vi "ExecuteMenuCommand.vi"(0 "reference":refnum<class "PackageNode.lvclass">, 1 "Command":string, 5 "error in (no error)":errorcluster) -> (14 "reference out":refnum<class "PackageNode.lvclass">, 15 "EditorAction":T3, 16 "FlattenCommandSettings":T1, 19 "error out":errorcluster)   [LabVIEW 2020, in "PackageNode.lvclass"]
uses:
  <resource>/Framework/Providers/Open_GDS/UML/PackageNode_class/PackageNode.lvclass
  C:/Program Files (x86)/National Instruments/LabVIEW 2020/resource/Framework/Providers/Open_GDS/UML/RectangularNode_class/RectangularNode.lvclass
  C:/Program Files (x86)/National Instruments/LabVIEW 2020/resource/Framework/Providers/Open_GDS/UML/AbstractNode_class/AbstractNode.lvclass
  <resource>/Framework/Providers/Open_GDS/UML/UMLEditor/UMLEditor EditorActionType.ctl
  <resource>/Framework/Providers/Open_GDS/UML/UMLEditor/UMLEditor FlattenCommandType.ctl
  <resource>/Framework/Providers/Open_GDS/UML/UMLEditor/UMLEditor ExecuteCommandType.ctl
  <resource>/Framework/Providers/Open_GDS/UML/General/Rectangle/Rectangle Rectangle2D.ctl
  <resource>/Framework/Providers/Open_GDS/UML/AbstractNode_class/AbstractNode.lvclass
  <resource>/Framework/Providers/Open_GDS/UML/RectangularNode_class/RectangularNode.lvclass
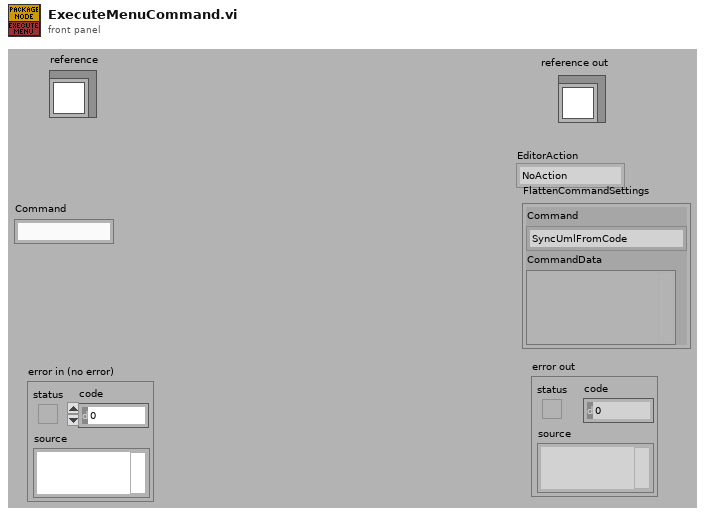
[diagram p1: front panel]
types:
  T1 = typedef "UMLEditor FlattenCommandType.ctl" = cluster{"Command":T2, "CommandData":variant}
  T2 = typedef "UMLEditor ExecuteCommandType.ctl" = enum16{"SyncUmlFromCode", "SyncCodeFromUML", "OpenClass", "OpenFile", "CreateClass", "CreateVI", "OpenClassAttribute", "LocateInProject", "GraphExecute"}
  T3 = typedef "UMLEditor EditorActionType.ctl" = enum16{"NoAction", "Repaint", "ExecuteCommand"}
  T4 = typedef "Rectangle Rectangle2D.ctl" = cluster{"x":dbl, "y":dbl, "width":dbl, "height":dbl}
  T5 = typedef "PackageNode.lvclass/ObjectAttributes.ctl" = cluster{"name":string, "contents":refnum<class "MultiLineString.lvclass">, "DEFAULT_TOP_WIDTH":i32, "DEFAULT_TOP_HEIGHT":i32, "DEFAULT_WIDTH":i32, "DEFAULT_HEIGHT":i32, "NAME_GAP":i32, "XGAP":i32, "YGAP":i32, "Collapsed":bool, "Note color":u32, "Justification":u16}
  T6 = typedef "AbstractNode.lvclass/ObjectAttributes.ctl" = cluster{"parent":refnum<class "AbstractNode.lvclass">, "children":refnum<class "AbstractNode.lvclass">[], "Hidden":bool}
  T7 = typedef "RectangularNode.lvclass/ObjectAttributes.ctl" = cluster{"bounds":T4}
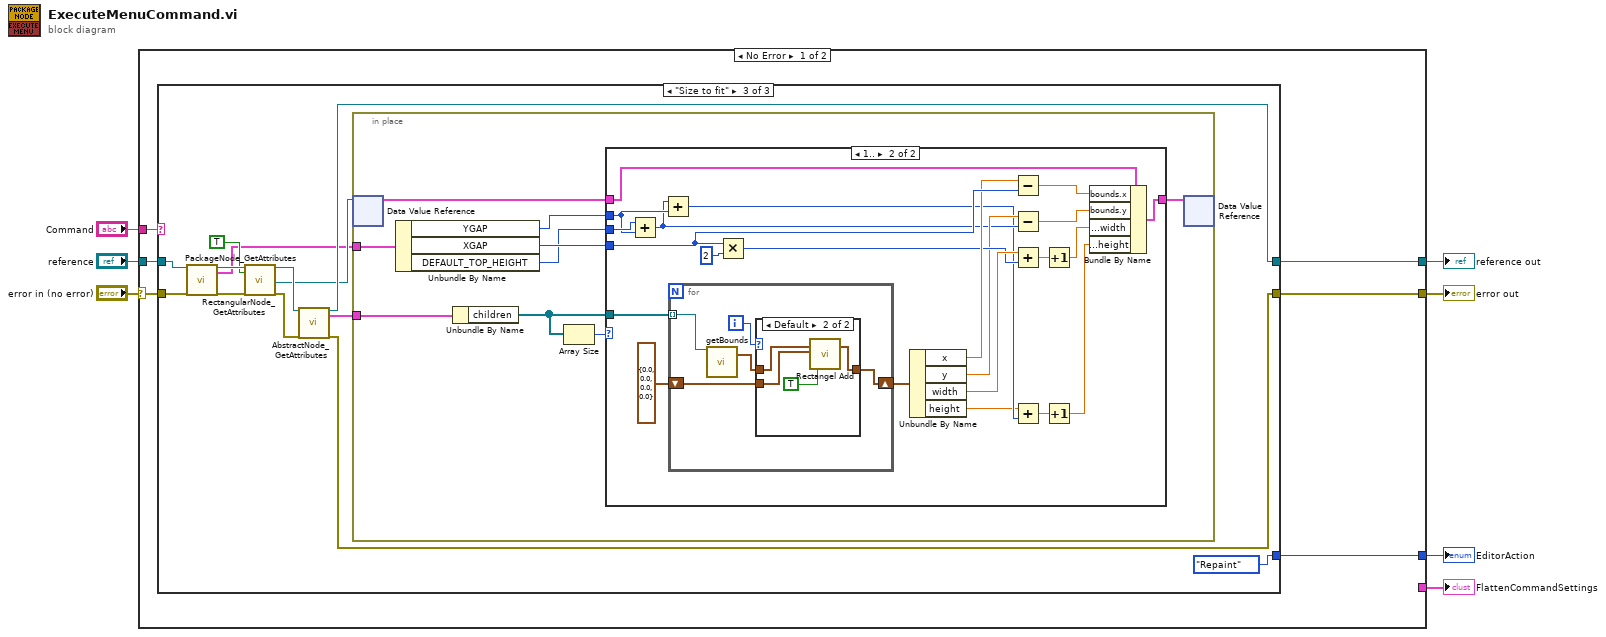
[diagram p0: block diagram]
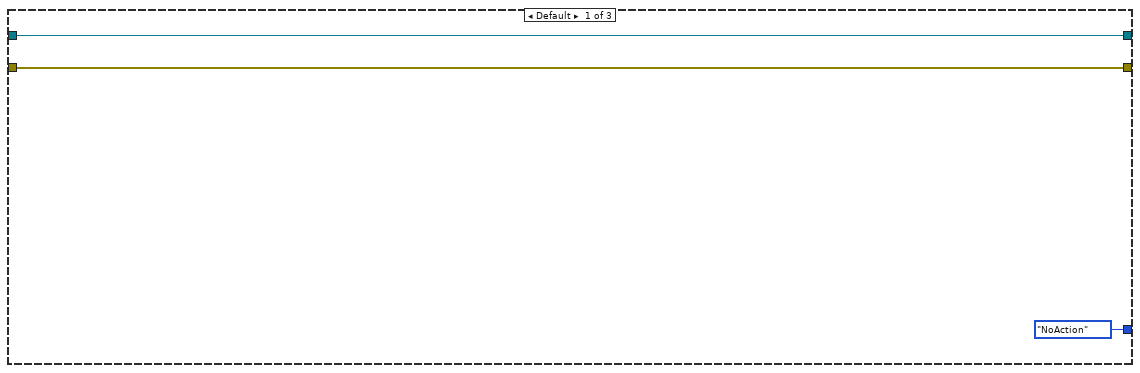
[diagram p2: hidden frame]
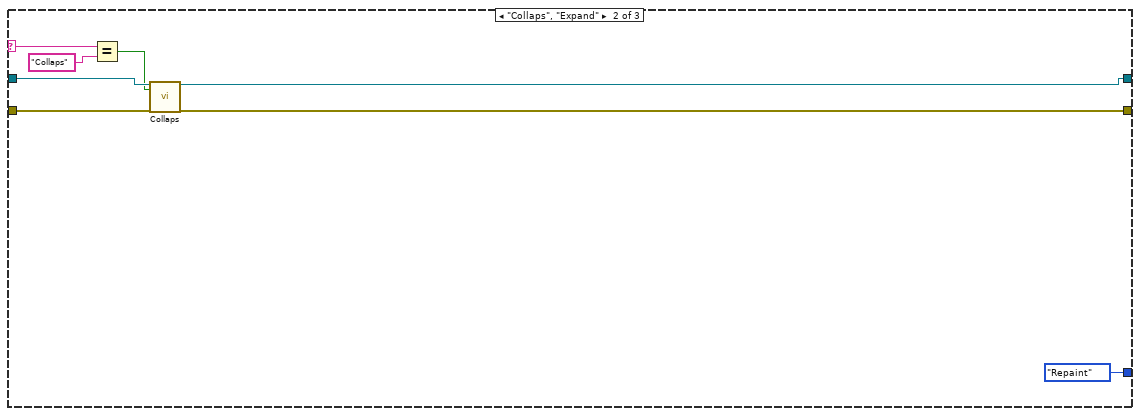
[diagram p3: hidden frame]
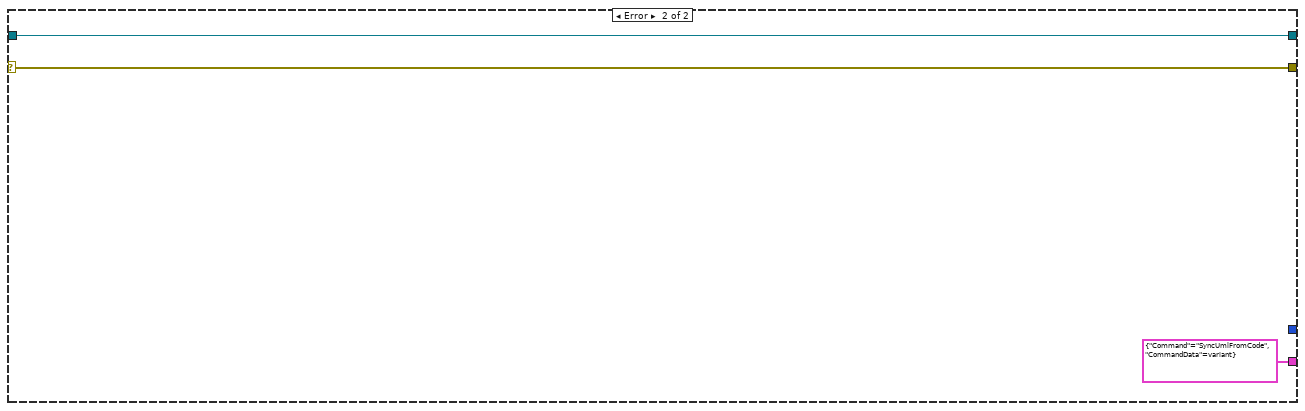
[diagram p6: hidden frame]
diagram:
  n1 = case shown="No Error" "error in (no error)" {
    selector: "error in (no error)" -> [w8 w81]
    tunnel: "reference" -> [w9 w82]
    tunnel: [w11 w81] -> w5
    tunnel: [w12 w82] -> w4
    tunnel: "Command" -> [w13 _]
    tunnel: [w10 _] -> w2
    tunnel: [_ T1 {"Command"=enum."SyncUmlFromCode", "CommandData"=variant} ("FlattenCommandSettings")] -> w1
    frame No Error {
      n2 = case shown="\"Size to fit\"" w13 {
        selector: w13 -> [_ w23 _]
        tunnel: w8 -> [w15 w19 w35]
        tunnel: w9 -> [w16 w21 w37]
        tunnel: [w16 w17 w36] -> w12
        tunnel: [w15 w18 w34] -> w11
        tunnel: [UMLEditor_EditorActionType."NoAction" ("EditorAction") UMLEditor_EditorActionType."Repaint" ("EditorAction") UMLEditor_EditorActionType."Repaint" ("EditorAction")] -> w10
        frame Default {
        }
        frame "Collaps", "Expand" {
          n3 = Equal?(x=w23, y="Collaps") -> (x = y?=w20:bool)
          n4 = call-dynamic "Collaps.vi"("reference in"=w21, "Collaps"=w20, "error in (no error)"=w19) -> ("reference out"=w17:refnum<class "PackageNode.lvclass">, "error out"=w18:errorcluster)  [unwired: 15 in]
        }
        frame "Size to fit" {
          n5 = call <resource>:"PackageNode_GetAttributes.vi"("reference in"=w37, "error in (no error)"=w35) -> ("reference out"=w32:refnum<class "PackageNode.lvclass">, "Data"=w25:T5, "error out"=w31:errorcluster)  [unwired: 14 in, 1 out]
          n6 = call <resource>:"RectangularNode_GetAttributes.vi"("reference in"=w32, "OnlyGetDvrReference(False)"=TRUE, "error in (no error)"=w31) -> ("reference out"=w30:refnum<class "PackageNode.lvclass">, "DataRef"=w28:refnum<data-value>, "error out"=w29:errorcluster)  [unwired: 13 in, 1 out]
          n7 = call <resource>:"AbstractNode_GetAttributes.vi"("reference in"=w30, "error in (no error)"=w29) -> ("reference out"=w36:refnum<class "PackageNode.lvclass">, "Data"=w26:T6, "error out"=w34:errorcluster)  [unwired: 14 in, 1 out]
          n8 = in-place {
            in-place-border: w26 -> [w41]
            in-place-border: w25 -> [w40]
            n9 = in-place-dvr #1(w28) -> (w43:T7)  [unwired: 1 out]
            n10 = Unbundle By Name(w40) -> ("YGAP"=w46:i32, "XGAP"=w45:i32, "DEFAULT_TOP_HEIGHT"=w44:i32)
            n11 = Unbundle By Name(w41) -> ("children"=w39:refnum<class "AbstractNode.lvclass">[])
            n12 = Array Size(array=w39) -> (size(s)=w38:i32)
            n13 = case shown="1.." w38 {
              tunnel: [w47 w69] -> w42
              tunnel: w45 -> [_ w68]
              tunnel: w44 -> [_ w67]
              tunnel: w46 -> [_ w66]
              tunnel: w39 -> [_ w65]
              tunnel: w43 -> [w47 w64]
              frame 0, Default {
              }
              frame 1.. {
                n14 = Add(x=w67, y=w66) -> (x+y=w53:i32)
                n15 = Add(x=w53, y=w66) -> (x+y=w52:i32)
                n16 = for {
                  tunnel: w65 -> [w74] mode=indexing
                  shift-right: [w72] -> w62
                  shift-left: T4 {"x"=0.0, "y"=0.0, "width"=0.0, "height"=0.0} ("bounds") -> [w70]
                  i -> [w73]
                  n17 = call-dynamic "getBounds.vi"("reference"=w74) -> ("bounds"=w71:T4)  [unwired: 16 in, 2 out]
                  n18 = case shown="Default" w73 {
                    tunnel: [w75 w77] -> w72
                    tunnel: w71 -> [w75 w78]
                    tunnel: w70 -> [_ w79]
                    frame 0 {
                    }
                    frame Default {
                      n19 = call <resource>:"Rectangel Add.vi"("bounds1"=w78, "bounds2"=w79, "useAbsoluteCordinates(False)"=TRUE) -> ("boundsAdded"=w77:T4)  [unwired: 15 in, 1 out]
                    }
                  }
                }
                n20 = Multiply(x=w68, y=2) -> (x*y=w57:i32)
                n21 = Unbundle By Name(w62) -> ("x"=w61:dbl, "y"=w56:dbl, "width"=w59:dbl, "height"=w51:dbl)
                n22 = Subtract(x=w61, y=w68) -> (x-y=w60:dbl)
                n23 = Subtract(x=w56, y=w53) -> (x-y=w55:dbl)
                n24 = Add(x=w59, y=w57) -> (x+y=w54:dbl)
                n25 = Add(x=w51, y=w52) -> (x+y=w50:dbl)
                n26 = Increment(x=w54) -> (x+1=w49:dbl)
                n27 = Increment(x=w50) -> (x+1=w48:dbl)
                n28 = Bundle By Name(cluster=w64, "bounds.x"=w60, "bounds.y"=w55, "bounds.width"=w49, "bounds.height"=w48) -> (w69:T7)
              }
            }
            n29 = in-place-dvr #1(w42) -> ()  [unwired: 2 out]
          }
        }
      }
    }
    frame Error {
    }
  }
  "reference out" <- w4
  "error out" <- w5
  "FlattenCommandSettings" <- w1
  "EditorAction" <- w2
